vi "Get Server Data.vi"(10 "Tag Data":T4[](array[typedef]), 11 "OPC UA Client in":T5) -> (1 "Browse Names":string[](array[string]), 2 "Tag Data":T4[](array[typedef]), 3 "OPC UA Client Refnum out":T5)   [LabVIEW 2018, in "OPC UA.lvlib"]
uses:
  OPC UA.lvlib
  <vilib>/OPCUA/controls/OPC UA Client Refnum.ctl
  <vilib>/OPCUA/controls/NodeId.ctl
  <vilib>/OPCUA/controls/Node Class.ctl
  OPC Tag Data.ctl
  <vilib>/OPCUA/controls/Read Variant Result.ctl
  <vilib>/OPCUA/controls/OPC UA StatusCode.ctl
  <vilib>/OPCUA/client/Multiple Read Variant.vi
  <vilib>/OPCUA/NI OPC UA Client.lvlib
  Variable Data Cluster.ctl
  Object Data Cluster.ctl
  <vilib>/regexp/Match Regular Expression.xnode
panel:
  out "results":T1[](array[typedef]) {"status" items=["Good"=0, "Good_SubscriptionTransferred"=2949120, "Good_CompletesAsynchronously"=3014656, "Good_Overload"=3080192, "Good_Clamped"=3145728, "Good_LocalOverride"=9830400, "Good_EntryInserted"=10616832, "Good_EntryReplaced"=10682368, "Good_NoData"=10813440, "Good_MoreData"=10878976, "Good_CommunicationEvent"=10944512, "Good_ShutdownEvent"=11010048, "Good_CallAgain"=11075584, "Good_NonCriticalTimeout"=11141120, "Good_ResultsMayBeIncomplete"=12189696, "Good_DataIgnored"=14221312, "Uncertain"=1073741824, "Uncertain_ReferenceOutOfServer"=1080819712, "Uncertain_NoCommunicationLastUsableValue"=1083113472, "Uncertain_LastUsableValue"=1083179008, "Uncertain_SubstituteValue"=1083244544, "Uncertain_InitialValue"=1083310080, "Uncertain_SensorNotAccurate"=1083375616, "Uncertain_EngineeringUnitsExceeded"=1083441152, "Uncertain_SubNormal"=1083506688, "Uncertain_DataSubNormal"=1084489728, "Uncertain_ReferenceNotDeleted"=1086062592, "Uncertain_NotAllNodesAvailable"=1086324736, "Bad"=2147483648, "Bad_UnexpectedError"=2147549184, "Bad_InternalError"=2147614720, "Bad_OutOfMemory"=2147680256, "Bad_ResourceUnavailable"=2147745792, "Bad_CommunicationError"=2147811328, "Bad_EncodingError"=2147876864, "Bad_DecodingError"=2147942400, "Bad_EncodingLimitsExceeded"=2148007936, "Bad_UnknownResponse"=2148073472, "Bad_Timeout"=2148139008, "Bad_ServiceUnsupported"=2148204544, "Bad_Shutdown"=2148270080, "Bad_ServerNotConnected"=2148335616, "Bad_ServerHalted"=2148401152, "Bad_NothingToDo"=2148466688, "Bad_TooManyOperations"=2148532224, "Bad_DataTypeIdUnknown"=2148597760, "Bad_CertificateInvalid"=2148663296, "Bad_SecurityChecksFailed"=2148728832, "Bad_CertificateTimeInvalid"=2148794368, "Bad_CertificateIssuerTimeInvalid"=2148859904, "Bad_CertificateHostNameInvalid"=2148925440, "Bad_CertificateUriInvalid"=2148990976, "Bad_CertificateUseNotAllowed"=2149056512, "Bad_CertificateIssuerUseNotAllowed"=2149122048, "Bad_CertificateUntrusted"=2149187584, "Bad_CertificateRevocationUnknown"=2149253120, "Bad_CertificateIssuerRevocationUnknown"=2149318656, "Bad_CertificateRevoked"=2149384192, "Bad_CertificateIssuerRevoked"=2149449728, "Bad_UserAccessDenied"=2149515264, "Bad_IdentityTokenInvalid"=2149580800, "Bad_IdentityTokenRejected"=2149646336, "Bad_SecureChannelIdInvalid"=2149711872, "Bad_InvalidTimestamp"=2149777408, "Bad_NonceInvalid"=2149842944, "Bad_SessionIdInvalid"=2149908480, "Bad_SessionClosed"=2149974016, "Bad_SessionNotActivated"=2150039552, "Bad_SubscriptionIdInvalid"=2150105088, "Bad_RequestHeaderInvalid"=2150236160, "Bad_TimestampsToReturnInvalid"=2150301696, "Bad_RequestCancelledByClient"=2150367232, "Bad_NoCommunication"=2150694912, "Bad_WaitingForInitialData"=2150760448, "Bad_NodeIdInvalid"=2150825984, "Bad_NodeIdUnknown"=2150891520, "Bad_AttributeIdInvalid"=2150957056, "Bad_IndexRangeInvalid"=2151022592, "Bad_IndexRangeNoData"=2151088128, "Bad_DataEncodingInvalid"=2151153664, "Bad_DataEncodingUnsupported"=2151219200, "Bad_NotReadable"=2151284736, "Bad_NotWritable"=2151350272, "Bad_OutOfRange"=2151415808, "Bad_NotSupported"=2151481344, "Bad_NotFound"=2151546880, "Bad_ObjectDeleted"=2151612416, "Bad_NotImplemented"=2151677952, "Bad_MonitoringModeInvalid"=2151743488, "Bad_MonitoredItemIdInvalid"=2151809024, "Bad_MonitoredItemFilterInvalid"=2151874560, "Bad_MonitoredItemFilterUnsupported"=2151940096, "Bad_FilterNotAllowed"=2152005632, "Bad_StructureMissing"=2152071168, "Bad_EventFilterInvalid"=2152136704, "Bad_ContentFilterInvalid"=2152202240, "Bad_FilterOperandInvalid"=2152267776, "Bad_ContinuationPointInvalid"=2152333312, "Bad_NoContinuationPoints"=2152398848, "Bad_ReferenceTypeIdInvalid"=2152464384, "Bad_BrowseDirectionInvalid"=2152529920, "Bad_NodeNotInView"=2152595456, "Bad_ServerUriInvalid"=2152660992, "Bad_ServerNameMissing"=2152726528, "Bad_DiscoveryUrlMissing"=2152792064, "Bad_SempahoreFileMissing"=2152857600, "Bad_RequestTypeInvalid"=2152923136, "Bad_SecurityModeRejected"=2152988672, "Bad_SecurityPolicyRejected"=2153054208, "Bad_TooManySessions"=2153119744, "Bad_UserSignatureInvalid"=2153185280, "Bad_ApplicationSignatureInvalid"=2153250816, "Bad_NoValidCertificates"=2153316352, "Bad_RequestCancelledByRequest"=2153381888, "Bad_ParentNodeIdInvalid"=2153447424, "Bad_ReferenceNotAllowed"=2153512960, "Bad_NodeIdRejected"=2153578496, "Bad_NodeIdExists"=2153644032, "Bad_NodeClassInvalid"=2153709568, "Bad_BrowseNameInvalid"=2153775104, "Bad_BrowseNameDuplicated"=2153840640, "Bad_NodeAttributesInvalid"=2153906176, "Bad_TypeDefinitionInvalid"=2153971712, "Bad_SourceNodeIdInvalid"=2154037248, "Bad_TargetNodeIdInvalid"=2154102784, "Bad_DuplicateReferenceNotAllowed"=2154168320, "Bad_InvalidSelfReference"=2154233856, "Bad_ReferenceLocalOnly"=2154299392, "Bad_NoDeleteRights"=2154364928, "Bad_ServerIndexInvalid"=2154430464, "Bad_ViewIdUnknown"=2154496000, "Bad_TooManyMatches"=2154627072, "Bad_QueryTooComplex"=2154692608, "Bad_NoMatch"=2154758144, "Bad_MaxAgeInvalid"=2154823680, "Bad_HistoryOperationInvalid"=2154889216, "Bad_HistoryOperationUnsupported"=2154954752, "Bad_WriteNotSupported"=2155020288, "Bad_TypeMismatch"=2155085824, "Bad_MethodInvalid"=2155151360, "Bad_ArgumentsMissing"=2155216896, "Bad_TooManySubscriptions"=2155282432, "Bad_TooManyPublishRequests"=2155347968, "Bad_NoSubscription"=2155413504, "Bad_SequenceNumberUnknown"=2155479040, "Bad_MessageNotAvailable"=2155544576, "Bad_InsufficientClientProfile"=2155610112, "Bad_TcpServerTooBusy"=2155675648, "Bad_TcpMessageTypeInvalid"=2155741184, "Bad_TcpSecureChannelUnknown"=2155806720, "Bad_TcpMessageTooLarge"=2155872256, "Bad_TcpNotEnoughResources"=2155937792, "Bad_TcpInternalError"=2156003328, "Bad_TcpEndpointUrlInvalid"=2156068864, "Bad_RequestInterrupted"=2156134400, "Bad_RequestTimeout"=2156199936, "Bad_SecureChannelClosed"=2156265472, "Bad_SecureChannelTokenUnknown"=2156331008, "Bad_SequenceNumberInvalid"=2156396544, "Bad_ConfigurationError"=2156462080, "Bad_NotConnected"=2156527616, "Bad_DeviceFailure"=2156593152, "Bad_SensorFailure"=2156658688, "Bad_OutOfService"=2156724224, "Bad_DeadbandFilterInvalid"=2156789760, "Bad_RefreshInProgress"=2157379584, "Bad_ConditionAlreadyDisabled"=2157445120, "Bad_ConditionDisabled"=2157510656, "Bad_EventIdUnknown"=2157576192, "Bad_NoData"=2157641728, "Bad_DataLost"=2157772800, "Bad_DataUnavailable"=2157838336, "Bad_EntryExists"=2157903872, "Bad_NoEntryExists"=2157969408, "Bad_TimestampNotSupported"=2158034944, "Bad_InvalidArgument"=2158690304, "Bad_ConnectionRejected"=2158755840, "Bad_Disconnect"=2158821376, "Bad_ConnectionClosed"=2158886912, "Bad_InvalidState"=2158952448, "Bad_EndOfStream"=2159017984, "Bad_NoDataAvailable"=2159083520, "Bad_WaitingForResponse"=2159149056, "Bad_OperationAbandoned"=2159214592, "Bad_ExpectedStreamToBlock"=2159280128, "Bad_WouldBlock"=2159345664, "Bad_SyntaxError"=2159411200, "Bad_MaxConnectionsReached"=2159476736, "Bad_RequestTooLarge"=2159542272, "Bad_ResponseTooLarge"=2159607808, "Bad_EventNotAcknowledgeable"=2159738880, "Bad_InvalidTimestampArgument"=2159869952, "Bad_ProtocolVersionUnsupported"=2159935488, "Bad_StateNotActive"=2160001024, "Bad_FilterOperatorInvalid"=2160132096, "Bad_FilterOperatorUnsupported"=2160197632, "Bad_FilterOperandCountMismatch"=2160263168, "Bad_FilterElementInvalid"=2160328704, "Bad_FilterLiteralInvalid"=2160394240, "Bad_IdentityChangeNotSupported"=2160459776, "Bad_NotTypeDefinition"=2160590848, "Bad_ViewTimestampInvalid"=2160656384, "Bad_ViewParameterMismatch"=2160721920, "Bad_ViewVersionInvalid"=2160787456, "Bad_ConditionAlreadyEnabled"=2160852992, "Bad_DialogNotActive"=2160918528, "Bad_DialogResponseInvalid"=2160984064, "Bad_ConditionBranchAlreadyAcked"=2161049600, "Bad_ConditionBranchAlreadyConfirmed"=2161115136, "Bad_ConditionAlreadyShelved"=2161180672, "Bad_ConditionNotShelved"=2161246208, "Bad_ShelvingTimeOutOfRange"=2161311744, "Bad_AggregateListMismatch"=2161377280, "Bad_AggregateNotSupported"=2161442816, "Bad_AggregateInvalidInputs"=2161508352, "Bad_BoundNotFound"=2161573888, "Bad_BoundNotSupported"=2161639424, "Bad_AggregateConfigurationRejected"=2161770496, "Bad_TooManyMonitoredItems"=2161836032]}
  out "browse result 2":T7(array[cluster]) {"node class" items=["Unspecified"=0, "Object"=1, "Variable"=2, "Method"=4, "Object Type"=8, "Variable Type"=16, "Reference Type"=32, "Data Type"=64, "View"=128]}
  out "OPC UA Client Refnum out 2":T5
  out "Browse Names 2":string[](array[string])
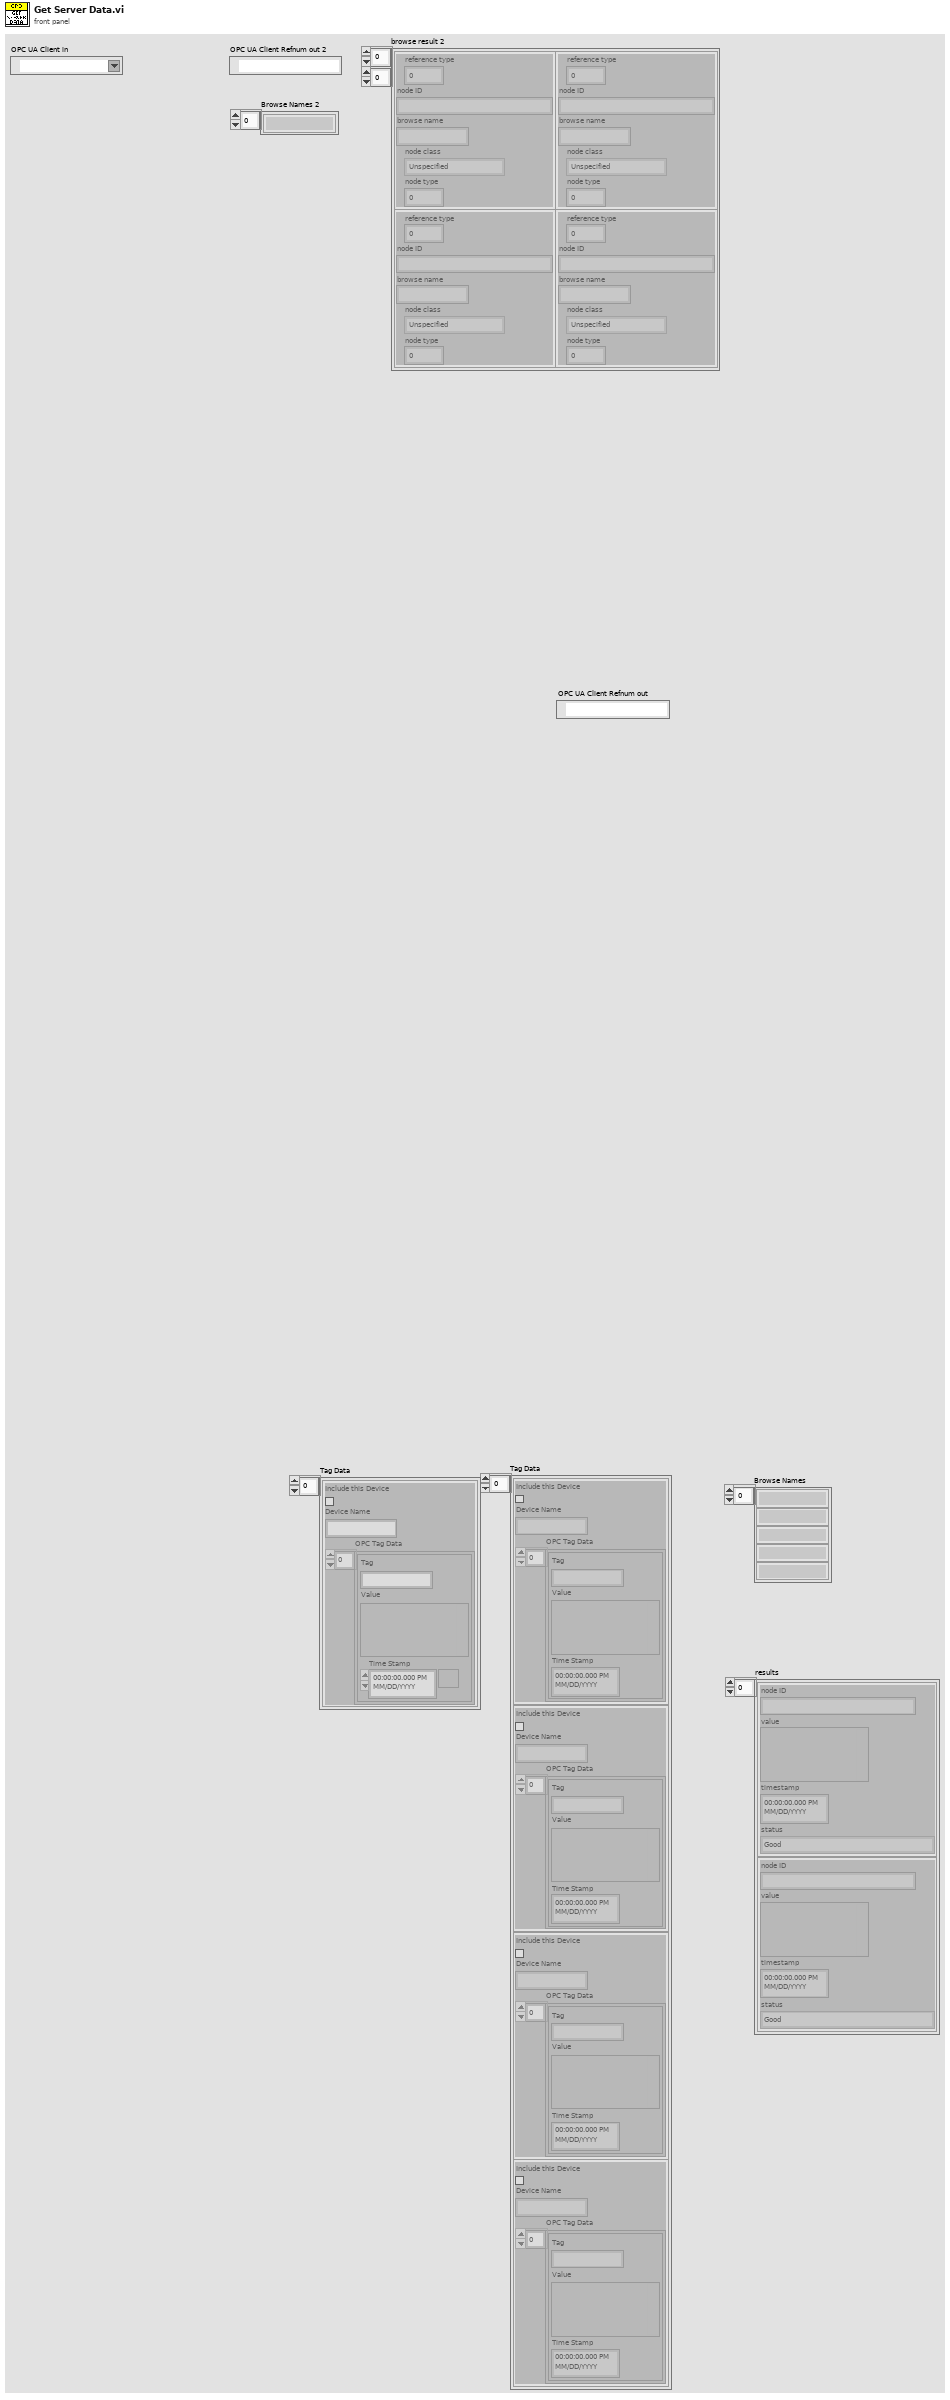
[diagram p1: front panel]
types:
  T1 = typedef "Read Variant Result.ctl" = cluster{"node ID":T2, "value ":variant, "timestamp":timestamp, "status":T3}
  T2 = typedef "NodeId.ctl" = string
  T3 = typedef "OPC UA StatusCode.ctl" = u32
  T4 = typedef "OPC UA.lvlib/OPC Tag Data.ctl" = cluster{"Include this Device":bool, "Device Name":string, "OPC Tag Data":cluster{"Tag":string, "Value":variant, "Time Stamp":timestamp}[]}
  T5 = typedef "OPC UA Client Refnum.ctl" = refnum<k21>
  T6 = typedef "Node Class.ctl" = u32
  T7 = cluster{"reference type":u32, "node ID":T2, "browse name":string, "node class":T6, "node type":u32}[][]
  T8 = typedef "OPC UA.lvlib/Object Data Cluster.ctl" = cluster{"Object Name":string, "Variable Array":T9[]}
  T9 = typedef "OPC UA.lvlib/Variable Data Cluster.ctl" = cluster{"node ID":T2, "browse name":string, "status":T3, "timestamp":timestamp, "value ":variant}
  T10 = cluster{"reference type":u32, "node ID":T2, "browse name":string, "node class":T6, "node type":u32}[]
  T11 = typedef "Data Type Indicator.ctl" = u16
  T12 = cluster{"name":string, "node class":u16, "data type":T11, "access":enum16{"Null", "Read", "Write", "Read&Write"}, "description":string}
  T13 = cluster{"Tag":string, "Value":variant, "Time Stamp":timestamp}[]
  T14 = cluster{"Tag":string, "Value":variant, "Time Stamp":timestamp}
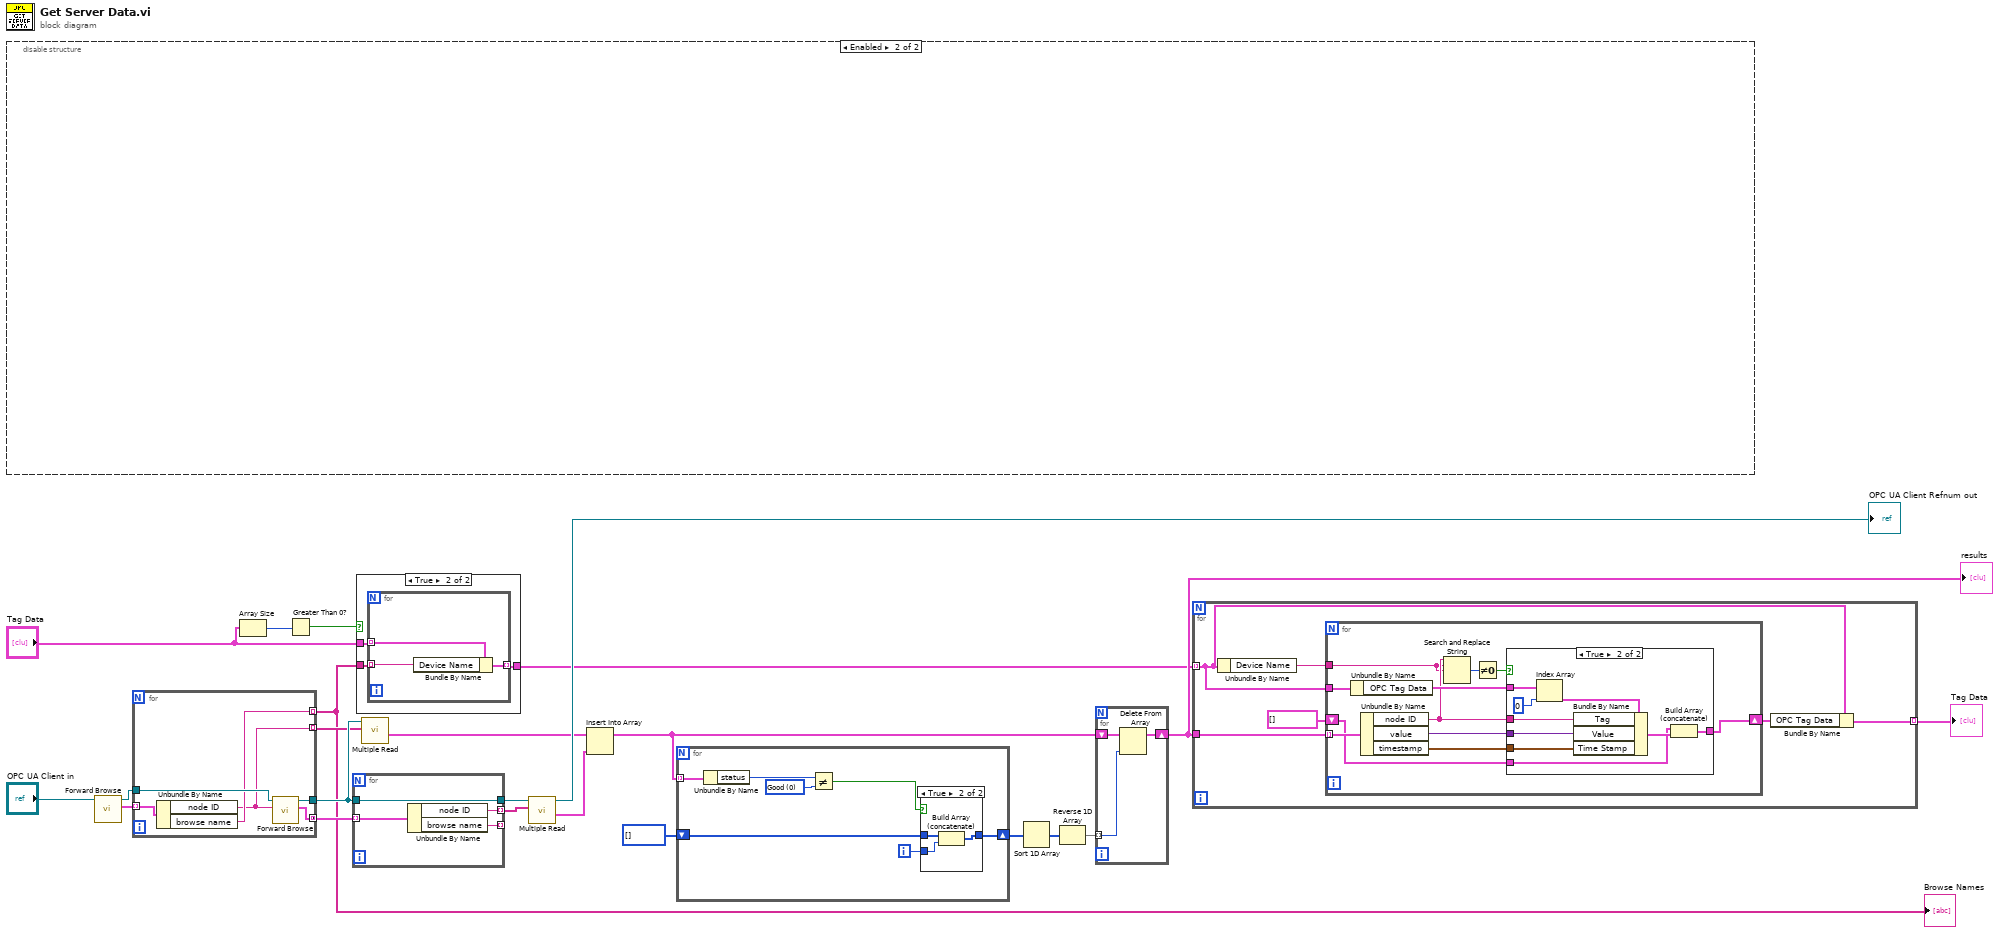
[diagram p0: block diagram]
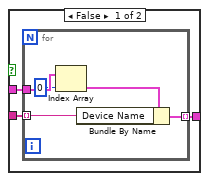
[diagram p2: hidden frame]
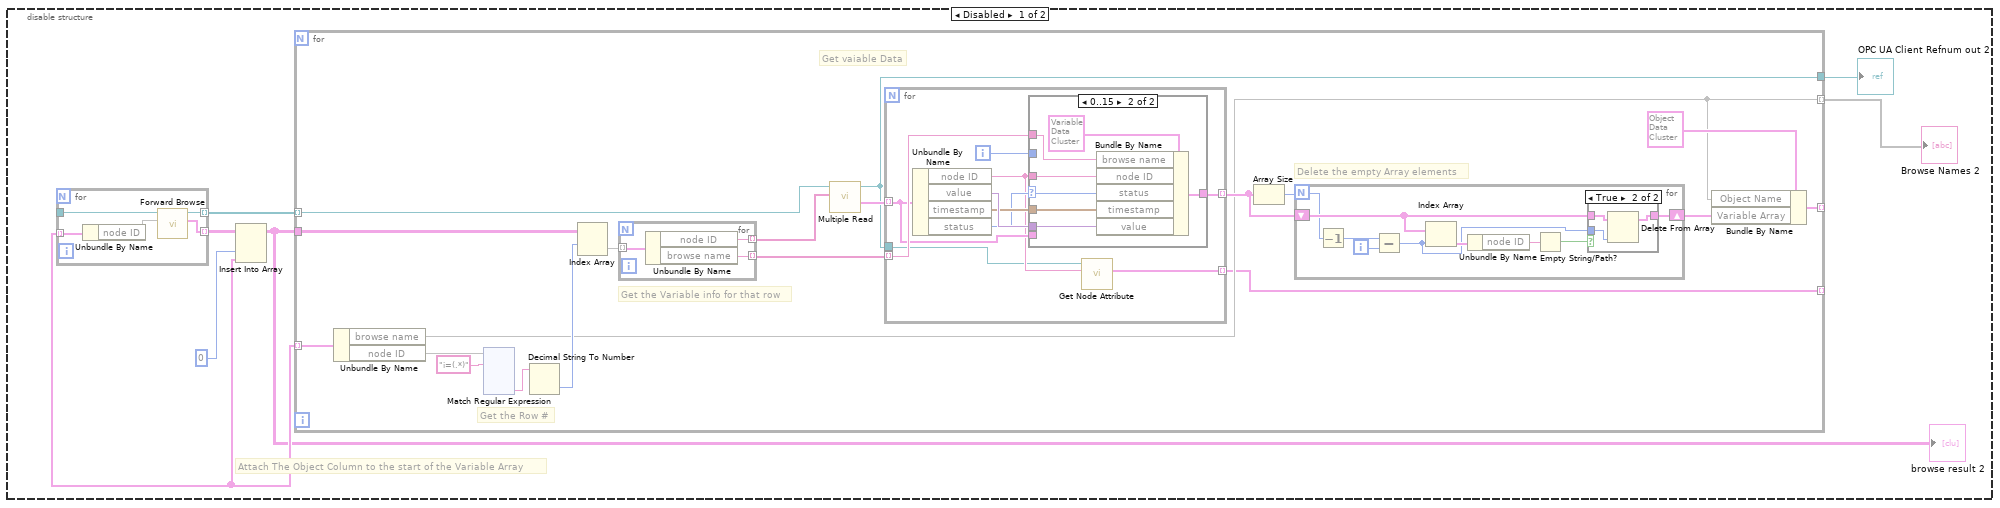
[diagram p5: hidden frame]
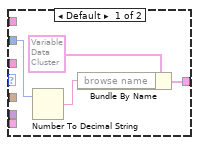
[diagram p7: hidden frame]
diagram:
  n1 = disable-structure shown="Enabled" {
    frame Disabled {
      # "Attach The Object Column to the start of the Variable Array"
      n2 = for {
        tunnel: w28 -> [w209] mode=indexing
        tunnel: _ -> [w208]
        tunnel: [w207] -> w29 mode=indexing
        tunnel: [w206] -> w27 mode=indexing
        n3 = Unbundle By Name(w209) -> ("node ID"=w205)
        n4 = call <vilib>:"Forward Browse.vi"("node ID"=w205, "OPC UA client refnum in"=w208) -> ("browse result"=w207:T10, "OPC UA client refnum out"=w206:T5)  [unwired: 6 in, 2 out]
      }
      n5 = Insert Into Array(array=w29, index (col)=0 ("disabled index (col)")) -> (w25:T7, new element=w28:T10)  [unwired: 1 in]
      "browse result 2" <- w25
      n6 = for {
        tunnel: w28 -> [w51] mode=indexing
        tunnel: [w49] -> w30 mode=indexing
        tunnel: w25 -> [w48]
        tunnel: w27 -> [w45] mode=indexing
        tunnel: [w35] -> w32 mode=indexing
        tunnel: [w34] -> w31
        tunnel: [w33] -> w24 mode=indexing
        # "Delete the empty Array elements"
        # "Get vaiable Data"
        # "Get the Variable info for that row"
        # "Get the Row #"
        n7 = Unbundle By Name(w51) -> ("browse name"=w35, "node ID"=w44)
        n8 = xnode "Match Regular Expression"("input string"=w44, "regular expression"="i=(.*)") -> ("submatch 1"=w42:string)  [unwired: 4 in, 5 out]
        n9 = Decimal String To Number(string=w42) -> (number=w47:i32)  [unwired: 2 in, 1 out]
        n10 = Index Array(array=w48, index (row)=w47) -> (element=w39:T10)  [unwired: 1 in]
        n11 = for {
          tunnel: w39 -> [w204] mode=indexing
          tunnel: [w203] -> w46 mode=indexing
          tunnel: [w202] -> w41 mode=indexing
          n12 = Unbundle By Name(w204) -> ("node ID"=w203:T2, "browse name"=w202:string)
        }
        n13 = call-poly <vilib>:"Multiple Read.vi"("node IDs"=w46, "OPC UA client refnum in"=w45) -> ("results"=w40:T1[], "OPC UA client refnum out"=w34:T5)  [unwired: 6 in, 2 out]
        n14 = for {
          tunnel: w40 -> [w70] mode=indexing
          tunnel: [w72] -> w37 mode=indexing
          tunnel: w41 -> [w71] mode=indexing
          tunnel: w34 -> [w66]
          tunnel: [w65] -> w33 mode=indexing
          i -> [w68]
          n15 = Unbundle By Name(w70) -> ("node ID"=w67:T2, "value"=w74:variant, "timestamp"=w73:timestamp, "status"=w69:T3)
          n16 = case shown="0..15" w69 {
            selector: w69 -> [_ w79]
            tunnel: w67 -> [_ w84]
            tunnel: w74 -> [_ w83]
            tunnel: w73 -> [_ w82]
            tunnel: [w77 w81] -> w72
            tunnel: w71 -> [_ w80]
            tunnel: w68 -> [w75 _]
            tunnel: w70 -> [_ _]
            frame Default {
              n17 = Number To Decimal String(number=w75) -> (decimal integer string=w76:string)  [unwired: 1 in]
              n18 = Bundle By Name(cluster=T9 {"node ID"="", "browse name"="Bad", "status"=2147483648, "timestamp"=timestamp(0 s since 1904-01-01), "value "=variant} ("Cluster"), "browse name"=w76) -> (w77:T9)
            }
            frame 0..15 {
              n19 = Bundle By Name(cluster=T9 {"node ID"="", "browse name"="", "status"=0, "timestamp"=timestamp(0 s since 1904-01-01), "value "=variant} ("Cluster"), "browse name"=w80, "node ID"=w84, "status"=w79, "timestamp"=w82, "value"=w83) -> (w81:T9)
            }
          }
          n20 = call <vilib>:"Get Node Attribute.vi"("node ID"=w67, "OPC UA client refnum in"=w66) -> ("node attribute"=w65:T12)  [unwired: 6 in, 3 out]
        }
        n21 = Array Size(array=w37) -> (size(s)=w36:i32)
        n22 = for {
          N: w36 -> [w53]
          shift-right: [w60] -> w38
          shift-left: w37 -> [w59]
          i -> [w55]
          n23 = Decrement(x=w53) -> (x-1=w52:i32)
          n24 = Subtract(x=w52, y=w55) -> (x-y=w54:i32)
          n25 = Index Array(array=w59, index=w54) -> (element=w58:T9)
          n26 = Unbundle By Name(w58) -> ("node ID"=w57:T2)
          n27 = Empty String/Path?(string/path=w57) -> (empty?=w56:bool)
          n28 = case shown="True" w56 {
            tunnel: [w61 w64] -> w60
            tunnel: w59 -> [w61 w63]
            tunnel: w54 -> [_ w62]
            frame False {
            }
            frame True {
              n29 = Delete From Array(array=w63, index=w62) -> (array with subset deleted=w64:T9[])  [unwired: 1 in, 1 out]
            }
          }
        }
        n30 = Bundle By Name(cluster=T8 {"Object Name"="", "Variable Array"=[{"node ID"="", "browse name"="", "status"=0, "timestamp"=timestamp(0 s since 1904-01-01), "value "=variant}]} ("Object Data"), "Object Name"=w35, "Variable Array"=w38) -> (w49:T8)
      }
      "Browse Names 2" <- w32
      "OPC UA Client Refnum out 2" <- w31
    }
    frame Enabled {
    }
  }
  n31 = call <vilib>:"Forward Browse.vi"("OPC UA client refnum in"="OPC UA Client in") -> ("browse result"=w22:T10, "OPC UA client refnum out"=w21:T5)  [unwired: 7 in, 2 out]
  n32 = for {
    tunnel: w22 -> [w215] mode=indexing
    tunnel: w21 -> [w214]
    tunnel: [w213] -> w16
    tunnel: [w212] -> w18 mode=concatenating
    tunnel: [w211] -> w7 mode=indexing
    tunnel: [w210] -> w15 mode=indexing
    n33 = Unbundle By Name(w215) -> ("node ID"=w210:T2, "browse name"=w211:string)
    n34 = call <vilib>:"Forward Browse.vi"("node ID"=w210, "OPC UA client refnum in"=w214) -> ("browse result"=w212:T10, "OPC UA client refnum out"=w213:T5)  [unwired: 6 in, 2 out]
  }
  "Browse Names" <- w7
  n35 = Array Size(array="Tag Data") -> (size(s)=w2:i32)
  n36 = Greater Than 0?(x=w2) -> (x > 0?=w1:bool)
  n37 = for {
    tunnel: w16 -> [w218]
    tunnel: w18 -> [w219] mode=indexing
    tunnel: [w218] -> w19
    tunnel: [w216] -> w17 mode=indexing
    tunnel: [w217] -> _ mode=indexing
    n38 = Unbundle By Name(w219) -> ("node ID"=w216:T2, "browse name"=w217:string)
  }
  n39 = case shown="True" w1 {
    tunnel: w7 -> [w222 w228]
    tunnel: [w221 w229] -> w5
    tunnel: "Tag Data" -> [w220 w230]
    frame False {
      n40 = for {
        tunnel: [w227] -> w221 mode=indexing
        tunnel: w222 -> [w226] mode=indexing
        tunnel: w220 -> [w225]
        n41 = Index Array(array=w225, index=0) -> (element=w224:T4)
        n42 = Bundle By Name(cluster=w224, "Device Name"=w226) -> (w227:T4)
      }
    }
    frame True {
      n43 = for {
        tunnel: [w233] -> w229 mode=indexing
        tunnel: w228 -> [w232] mode=indexing
        tunnel: w230 -> [w231] mode=indexing
        n44 = Bundle By Name(cluster=w231, "Device Name"=w232) -> (w233:T4)
      }
    }
  }
  n45 = call-poly <vilib>:"Multiple Read.vi"("node IDs"=w15, "OPC UA client refnum in"=w16) -> ("results"=w14:T1[])  [unwired: 6 in, 3 out]
  n46 = call-poly <vilib>:"Multiple Read.vi"("node IDs"=w17, "OPC UA client refnum in"=w19) -> ("results"=w13:T1[], "OPC UA client refnum out"=→"OPC UA Client Refnum out":T5)  [unwired: 6 in, 2 out]
  n47 = Insert Into Array(array=w14, new element=w13) -> (w8:T1[])  [unwired: 1 in]
  n48 = for {
    tunnel: w8 -> [w240] mode=indexing
    shift-right: [w236] -> w9
    shift-left: i32[] [] -> [w235]
    i -> [w237]
    w238 = T3 0 items=["Good"=0, "Good_SubscriptionTransferred"=2949120, "Good_CompletesAsynchronously"=3014656, "Good_Overload"=3080192, "Good_Clamped"=3145728, "Good_LocalOverride"=9830400, "Good_EntryInserted"=10616832, "Good_EntryReplaced"=10682368, "Good_NoData"=10813440, "Good_MoreData"=10878976, "Good_CommunicationEvent"=10944512, "Good_ShutdownEvent"=11010048, "Good_CallAgain"=11075584, "Good_NonCriticalTimeout"=11141120, "Good_ResultsMayBeIncomplete"=12189696, "Good_DataIgnored"=14221312, "Uncertain"=1073741824, "Uncertain_ReferenceOutOfServer"=1080819712, "Uncertain_NoCommunicationLastUsableValue"=1083113472, "Uncertain_LastUsableValue"=1083179008, "Uncertain_SubstituteValue"=1083244544, "Uncertain_InitialValue"=1083310080, "Uncertain_SensorNotAccurate"=1083375616, "Uncertain_EngineeringUnitsExceeded"=1083441152, "Uncertain_SubNormal"=1083506688, "Uncertain_DataSubNormal"=1084489728, "Uncertain_ReferenceNotDeleted"=1086062592, "Uncertain_NotAllNodesAvailable"=1086324736, "Bad"=2147483648, "Bad_UnexpectedError"=2147549184, "Bad_InternalError"=2147614720, "Bad_OutOfMemory"=2147680256, "Bad_ResourceUnavailable"=2147745792, "Bad_CommunicationError"=2147811328, "Bad_EncodingError"=2147876864, "Bad_DecodingError"=2147942400, "Bad_EncodingLimitsExceeded"=2148007936, "Bad_UnknownResponse"=2148073472, "Bad_Timeout"=2148139008, "Bad_ServiceUnsupported"=2148204544, "Bad_Shutdown"=2148270080, "Bad_ServerNotConnected"=2148335616, "Bad_ServerHalted"=2148401152, "Bad_NothingToDo"=2148466688, "Bad_TooManyOperations"=2148532224, "Bad_DataTypeIdUnknown"=2148597760, "Bad_CertificateInvalid"=2148663296, "Bad_SecurityChecksFailed"=2148728832, "Bad_CertificateTimeInvalid"=2148794368, "Bad_CertificateIssuerTimeInvalid"=2148859904, "Bad_CertificateHostNameInvalid"=2148925440, "Bad_CertificateUriInvalid"=2148990976, "Bad_CertificateUseNotAllowed"=2149056512, "Bad_CertificateIssuerUseNotAllowed"=2149122048, "Bad_CertificateUntrusted"=2149187584, "Bad_CertificateRevocationUnknown"=2149253120, "Bad_CertificateIssuerRevocationUnknown"=2149318656, "Bad_CertificateRevoked"=2149384192, "Bad_CertificateIssuerRevoked"=2149449728, "Bad_UserAccessDenied"=2149515264, "Bad_IdentityTokenInvalid"=2149580800, "Bad_IdentityTokenRejected"=2149646336, "Bad_SecureChannelIdInvalid"=2149711872, "Bad_InvalidTimestamp"=2149777408, "Bad_NonceInvalid"=2149842944, "Bad_SessionIdInvalid"=2149908480, "Bad_SessionClosed"=2149974016, "Bad_SessionNotActivated"=2150039552, "Bad_SubscriptionIdInvalid"=2150105088, "Bad_RequestHeaderInvalid"=2150236160, "Bad_TimestampsToReturnInvalid"=2150301696, "Bad_RequestCancelledByClient"=2150367232, "Bad_NoCommunication"=2150694912, "Bad_WaitingForInitialData"=2150760448, "Bad_NodeIdInvalid"=2150825984, "Bad_NodeIdUnknown"=2150891520, "Bad_AttributeIdInvalid"=2150957056, "Bad_IndexRangeInvalid"=2151022592, "Bad_IndexRangeNoData"=2151088128, "Bad_DataEncodingInvalid"=2151153664, "Bad_DataEncodingUnsupported"=2151219200, "Bad_NotReadable"=2151284736, "Bad_NotWritable"=2151350272, "Bad_OutOfRange"=2151415808, "Bad_NotSupported"=2151481344, "Bad_NotFound"=2151546880, "Bad_ObjectDeleted"=2151612416, "Bad_NotImplemented"=2151677952, "Bad_MonitoringModeInvalid"=2151743488, "Bad_MonitoredItemIdInvalid"=2151809024, "Bad_MonitoredItemFilterInvalid"=2151874560, "Bad_MonitoredItemFilterUnsupported"=2151940096, "Bad_FilterNotAllowed"=2152005632, "Bad_StructureMissing"=2152071168, "Bad_EventFilterInvalid"=2152136704, "Bad_ContentFilterInvalid"=2152202240, "Bad_FilterOperandInvalid"=2152267776, "Bad_ContinuationPointInvalid"=2152333312, "Bad_NoContinuationPoints"=2152398848, "Bad_ReferenceTypeIdInvalid"=2152464384, "Bad_BrowseDirectionInvalid"=2152529920, "Bad_NodeNotInView"=2152595456, "Bad_ServerUriInvalid"=2152660992, "Bad_ServerNameMissing"=2152726528, "Bad_DiscoveryUrlMissing"=2152792064, "Bad_SempahoreFileMissing"=2152857600, "Bad_RequestTypeInvalid"=2152923136, "Bad_SecurityModeRejected"=2152988672, "Bad_SecurityPolicyRejected"=2153054208, "Bad_TooManySessions"=2153119744, "Bad_UserSignatureInvalid"=2153185280, "Bad_ApplicationSignatureInvalid"=2153250816, "Bad_NoValidCertificates"=2153316352, "Bad_RequestCancelledByRequest"=2153381888, "Bad_ParentNodeIdInvalid"=2153447424, "Bad_ReferenceNotAllowed"=2153512960, "Bad_NodeIdRejected"=2153578496, "Bad_NodeIdExists"=2153644032, "Bad_NodeClassInvalid"=2153709568, "Bad_BrowseNameInvalid"=2153775104, "Bad_BrowseNameDuplicated"=2153840640, "Bad_NodeAttributesInvalid"=2153906176, "Bad_TypeDefinitionInvalid"=2153971712, "Bad_SourceNodeIdInvalid"=2154037248, "Bad_TargetNodeIdInvalid"=2154102784, "Bad_DuplicateReferenceNotAllowed"=2154168320, "Bad_InvalidSelfReference"=2154233856, "Bad_ReferenceLocalOnly"=2154299392, "Bad_NoDeleteRights"=2154364928, "Bad_ServerIndexInvalid"=2154430464, "Bad_ViewIdUnknown"=2154496000, "Bad_TooManyMatches"=2154627072, "Bad_QueryTooComplex"=2154692608, "Bad_NoMatch"=2154758144, "Bad_MaxAgeInvalid"=2154823680, "Bad_HistoryOperationInvalid"=2154889216, "Bad_HistoryOperationUnsupported"=2154954752, "Bad_WriteNotSupported"=2155020288, "Bad_TypeMismatch"=2155085824, "Bad_MethodInvalid"=2155151360, "Bad_ArgumentsMissing"=2155216896, "Bad_TooManySubscriptions"=2155282432, "Bad_TooManyPublishRequests"=2155347968, "Bad_NoSubscription"=2155413504, "Bad_SequenceNumberUnknown"=2155479040, "Bad_MessageNotAvailable"=2155544576, "Bad_InsufficientClientProfile"=2155610112, "Bad_TcpServerTooBusy"=2155675648, "Bad_TcpMessageTypeInvalid"=2155741184, "Bad_TcpSecureChannelUnknown"=2155806720, "Bad_TcpMessageTooLarge"=2155872256, "Bad_TcpNotEnoughResources"=2155937792, "Bad_TcpInternalError"=2156003328, "Bad_TcpEndpointUrlInvalid"=2156068864, "Bad_RequestInterrupted"=2156134400, "Bad_RequestTimeout"=2156199936, "Bad_SecureChannelClosed"=2156265472, "Bad_SecureChannelTokenUnknown"=2156331008, "Bad_SequenceNumberInvalid"=2156396544, "Bad_ConfigurationError"=2156462080, "Bad_NotConnected"=2156527616, "Bad_DeviceFailure"=2156593152, "Bad_SensorFailure"=2156658688, "Bad_OutOfService"=2156724224, "Bad_DeadbandFilterInvalid"=2156789760, "Bad_RefreshInProgress"=2157379584, "Bad_ConditionAlreadyDisabled"=2157445120, "Bad_ConditionDisabled"=2157510656, "Bad_EventIdUnknown"=2157576192, "Bad_NoData"=2157641728, "Bad_DataLost"=2157772800, "Bad_DataUnavailable"=2157838336, "Bad_EntryExists"=2157903872, "Bad_NoEntryExists"=2157969408, "Bad_TimestampNotSupported"=2158034944, "Bad_InvalidArgument"=2158690304, "Bad_ConnectionRejected"=2158755840, "Bad_Disconnect"=2158821376, "Bad_ConnectionClosed"=2158886912, "Bad_InvalidState"=2158952448, "Bad_EndOfStream"=2159017984, "Bad_NoDataAvailable"=2159083520, "Bad_WaitingForResponse"=2159149056, "Bad_OperationAbandoned"=2159214592, "Bad_ExpectedStreamToBlock"=2159280128, "Bad_WouldBlock"=2159345664, "Bad_SyntaxError"=2159411200, "Bad_MaxConnectionsReached"=2159476736, "Bad_RequestTooLarge"=2159542272, "Bad_ResponseTooLarge"=2159607808, "Bad_EventNotAcknowledgeable"=2159738880, "Bad_InvalidTimestampArgument"=2159869952, "Bad_ProtocolVersionUnsupported"=2159935488, "Bad_StateNotActive"=2160001024, "Bad_FilterOperatorInvalid"=2160132096, "Bad_FilterOperatorUnsupported"=2160197632, "Bad_FilterOperandCountMismatch"=2160263168, "Bad_FilterElementInvalid"=2160328704, "Bad_FilterLiteralInvalid"=2160394240, "Bad_IdentityChangeNotSupported"=2160459776, "Bad_NotTypeDefinition"=2160590848, "Bad_ViewTimestampInvalid"=2160656384, "Bad_ViewParameterMismatch"=2160721920, "Bad_ViewVersionInvalid"=2160787456, "Bad_ConditionAlreadyEnabled"=2160852992, "Bad_DialogNotActive"=2160918528, "Bad_DialogResponseInvalid"=2160984064, "Bad_ConditionBranchAlreadyAcked"=2161049600, "Bad_ConditionBranchAlreadyConfirmed"=2161115136, "Bad_ConditionAlreadyShelved"=2161180672, "Bad_ConditionNotShelved"=2161246208, "Bad_ShelvingTimeOutOfRange"=2161311744, "Bad_AggregateListMismatch"=2161377280, "Bad_AggregateNotSupported"=2161442816, "Bad_AggregateInvalidInputs"=2161508352, "Bad_BoundNotFound"=2161573888, "Bad_BoundNotSupported"=2161639424, "Bad_AggregateConfigurationRejected"=2161770496, "Bad_TooManyMonitoredItems"=2161836032] ("y")
    n49 = Unbundle By Name(w240) -> ("status"=w239:T3)
    n50 = Not Equal?(x=w239, y=w238) -> (x != y?=w234:bool)
    n51 = case shown="True" w234 {
      tunnel: w237 -> [_ w244]
      tunnel: [w241 w243] -> w236
      tunnel: w235 -> [w241 w242]
      frame False {
      }
      frame True {
        n52 = Build Array (concatenate)(w242, w244) -> (w243:i32[])
      }
    }
  }
  n53 = Sort 1D Array(array=w9) -> (sorted array=w11:i32[])
  n54 = Reverse 1D Array(array=w11) -> (reversed array=w10:i32[])
  n55 = for {
    tunnel: w10 -> [w246] mode=indexing
    shift-right: [w245] -> w6
    shift-left: w8 -> [w247]
    n56 = Delete From Array(array=w247, index=w246) -> (array with subset deleted=w245:T1[])  [unwired: 1 in, 1 out]
  }
  "results" <- w6
  n57 = for {
    tunnel: w6 -> [w253]
    tunnel: w5 -> [w251] mode=indexing
    tunnel: [w249] -> w4 mode=indexing
    n58 = Unbundle By Name(w251) -> ("Device Name"=w252:string)
    n59 = for {
      tunnel: w253 -> [w264] mode=indexing
      tunnel: w252 -> [w256]
      tunnel: w251 -> [w257]
      shift-right: [w255] -> w250
      shift-left: T13 [] -> [w254]
      n60 = Unbundle By Name(w257) -> ("OPC Tag Data"=w261:T13)
      n61 = Unbundle By Name(w264) -> ("node ID"=w260:T2, "value"=w259:variant, "timestamp"=w258:timestamp)
      n62 = Search and Replace String(input string=w260, search string=w256, replace string=w256) -> (number of replacements=w263:i32)  [unwired: 5 in, 3 out]
      n63 = Not Equal To 0?(x=w263) -> (x != 0?=w262:bool)
      n64 = case shown="True" w262 {
        tunnel: w261 -> [_ w270]
        tunnel: w260 -> [_ w274]
        tunnel: w259 -> [_ w273]
        tunnel: w258 -> [_ w272]
        tunnel: [w265 w268] -> w255
        tunnel: w254 -> [w265 w267]
        frame False {
        }
        frame True {
          n65 = Index Array(array=w270, index=0) -> (element=w271:T14)
          n66 = Bundle By Name(cluster=w271, "Tag"=w274, "Value"=w273, "Time Stamp"=w272) -> (w269:T14)
          n67 = Build Array (concatenate)(w267, w269) -> (w268:T13)
        }
      }
    }
    n68 = Bundle By Name(cluster=w251, "OPC Tag Data"=w250) -> (w249:T4)
  }
  "Tag Data" <- w4
